vi "Main.vi"(11 "Module Admin":refnum<class "Delacor_lib_QMH_Module Admin.lvclass">) -> ()   [LabVIEW 2020, in "AO DC.lvlib"]
doc: "This template is based off of the Queued Message Handler design pattern and the Queued Message Handler project template that ships with LabVIEW.\n\nThe main difference is that the queue is private to this module and communication between modules is performed via Broadcast and Request events.\n\nRequest events are wrapped in public API methods and are handled in the Event Handling Loop (EHL) of this VI. Any module can register for Broadcast events sent by this module. The EHL generates messages based on user interface actions.\n\nThe Message Handling Loop (MHL) processes messages generated by the EHL, or by other messages. The messages are string values, so new messages can be added easily to the Message Cases case structure in the MHL. Each message cluster can also provide an optional value for Message Data, which is a variant that can be converted to whatever message-specific data is required.\n_____\nBased on DQMH Project Template 6.1.0.94."
uses:
  AO DC.lvlib
  <vilib>/Delacor/Delacor QMH/Libraries/Module Admin_class/Delacor_lib_QMH_Module Admin.lvclass
  Module Data--cluster.ctl
  <vilib>/Delacor/Delacor QMH/Libraries/Message Queue_class/Delacor_lib_QMH_Message Queue.lvclass/Delacor_lib_QMH_Message Queue.ctl
  Stop Argument--cluster.ctl
  <vilib>/Delacor/Delacor QMH/Libraries/Module Admin_class/Delacor_lib_QMH_Module Admin.lvclass/Delacor_lib_QMH_Module Admin.ctl
  AO DC Init Argument--cluster.ctl
  AO DC Start Argument--cluster.ctl
  <vilib>/Utility/miscctls.llb/LVPointTypeDef.ctl
  <vilib>/Delacor/Delacor QMH/Libraries/Message Queue_class/Delacor_lib_QMH_Enqueue Message (Single).vi
  <vilib>/Delacor/Delacor QMH/Libraries/Module Admin_class/Delacor_lib_QMH_Get External Launch.vi
  <vilib>/DAQmx/write.llb/DAQmx Write (Analog DBL 1Chan 1Samp).vi
  <vilib>/Utility/error.llb/Error Cluster From Error Code.vi
  <vilib>/DAQmx/miscellaneous.llb/DAQmx Fill In Error Info.vi
  <vilib>/ErrorRing/Error Ring.xnode
  <vilib>/Delacor/Delacor QMH/Libraries/Message Queue_class/Delacor_lib_QMH_Message Queue.lvclass
panel:
  out "error out":errorcluster
  out "Status":string
  in  "Simulate MHL Error":bool
  in  "Simulate EHL Error":bool
  # "Other QMH Modules communicate with this Module via its Public API (wrappers for its Request Events).\n\nThis Module communicates with other Modules via its Broadcast Events.\nAny module that wants to get these messages, just registers for this module's Broadcast events."
  # "This template is for the Delacor Modified Queued Message Handler design pattern.\n\nSee the block diagram for more information on how to use this template."
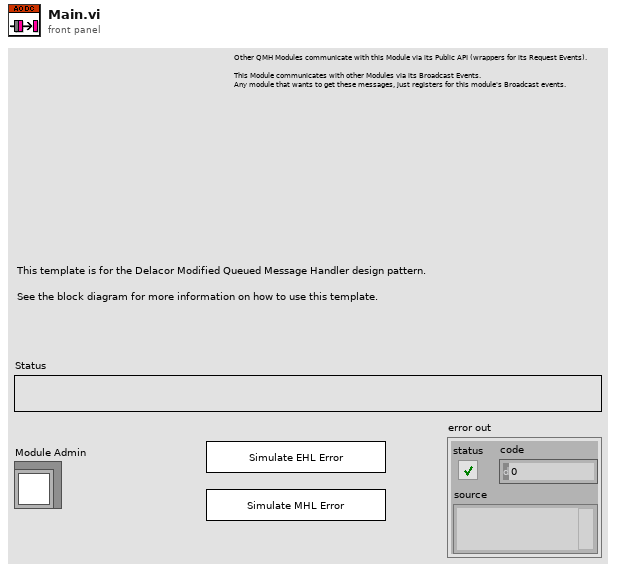
[diagram p1: front panel]
types:
  T1 = typedef "AO DC.lvlib/Request Events--cluster.ctl" = cluster{"Stop Module":refnum<user-event>, "Show Panel":refnum<user-event>, "Hide Panel":refnum<user-event>, "Get Module Execution Status":refnum<user-event>, "Show Diagram":refnum<user-event>, "AO DC Init":refnum<user-event>, "AO DC Start":refnum<user-event>}
  T2 = typedef "AO DC.lvlib/Module Data--cluster.ctl" = cluster{"Status":string, "AO DC Task":refnum<k21>, "User Value (Scaled)":dbl}
  T3 = enum32{"invalid lock state", "Not Locked", "Locked (No Password)", "Password-protected"}
  T4 = typedef "AO DC.lvlib/Stop Argument--cluster.ctl" = cluster{"Origin":string, "Exit via Stop Module Req?":bool, "Wait for Module to stop?":bool}
  T5 = typedef "AO DC.lvlib/AO DC Init Argument--cluster.ctl" = cluster{"AO DC Task":refnum<k21>, "User Value (Scaled)":dbl}
  T6 = typedef "AO DC.lvlib/AO DC Start Argument--cluster.ctl" = cluster{"Boolean":bool}
  T7 = typedef "LVPointTypeDef.ctl" = cluster{"Horizontal":i16, "Vertical":i16}
  T8 = enum32{"Invalid", "Standard", "Closed", "Hidden", "Minimized", "Maximized"}
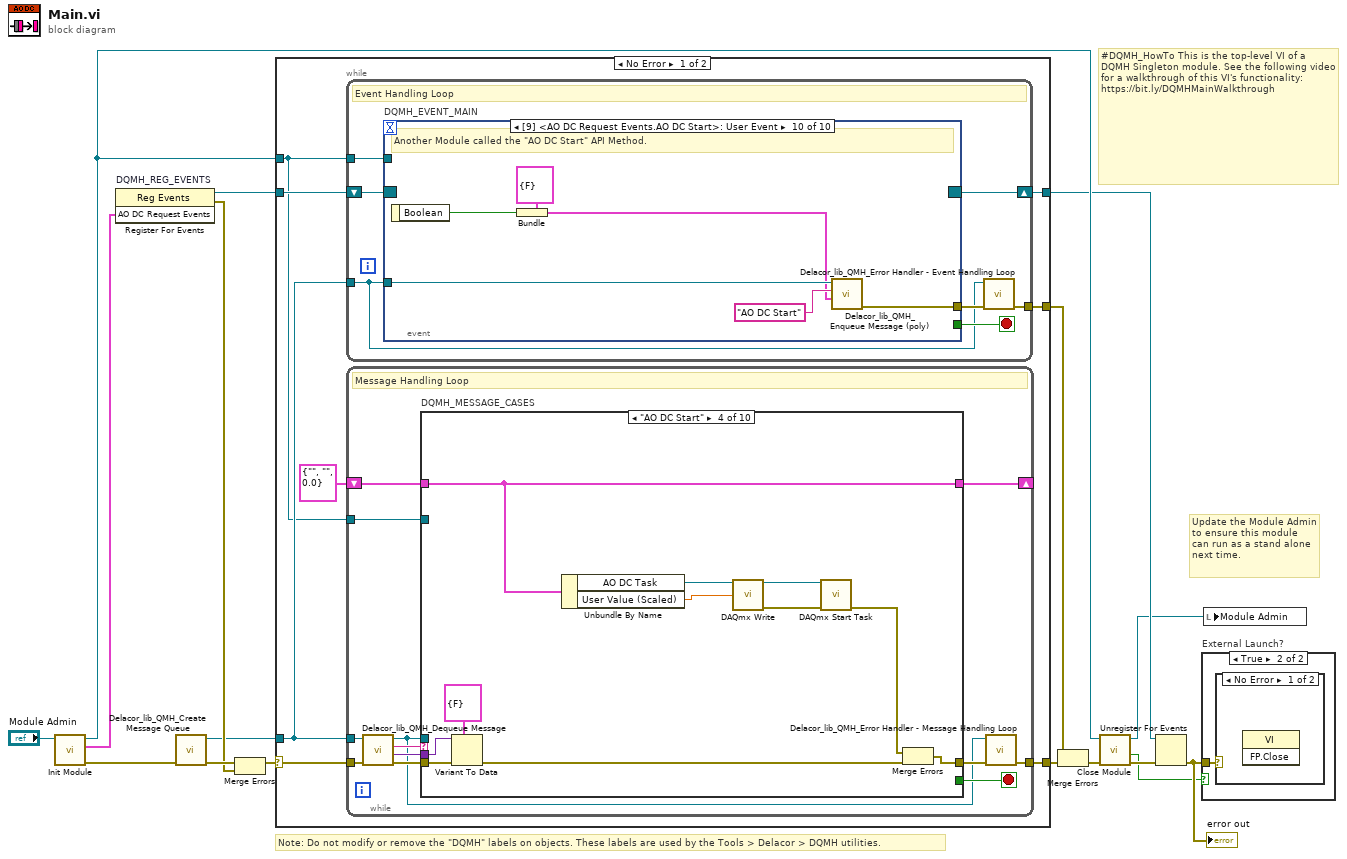
[diagram p0: block diagram]
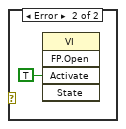
[diagram p3: hidden frame]
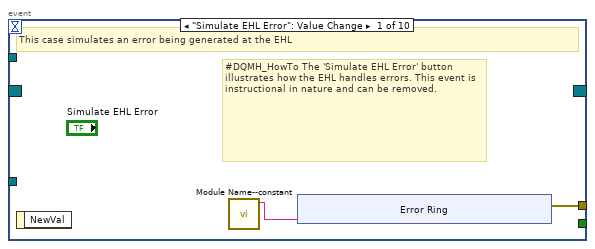
[diagram p4: hidden frame]
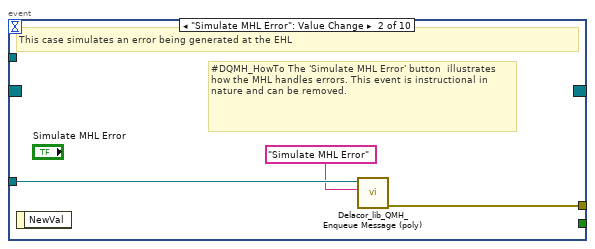
[diagram p5: hidden frame]
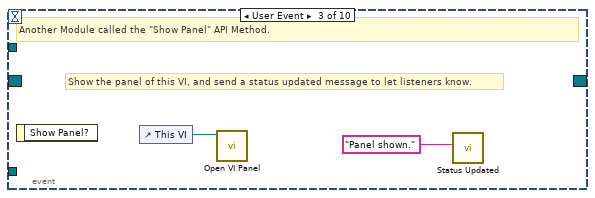
[diagram p6: hidden frame]
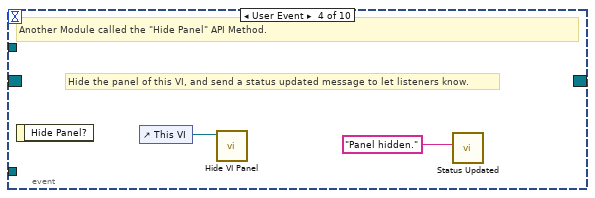
[diagram p7: hidden frame]
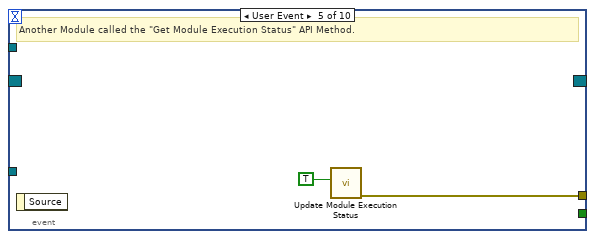
[diagram p8: hidden frame]
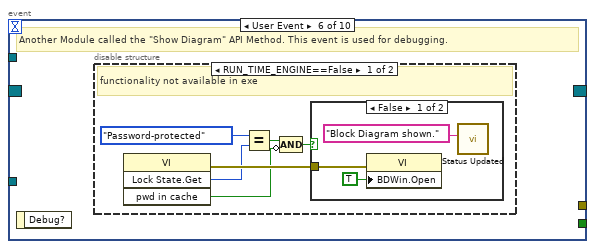
[diagram p9: hidden frame]
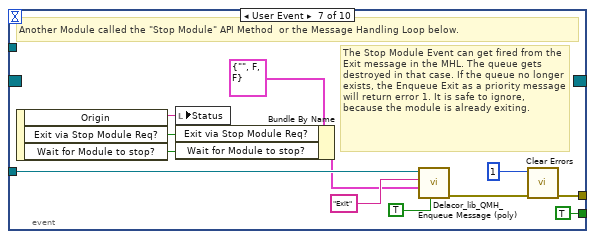
[diagram p12: hidden frame]
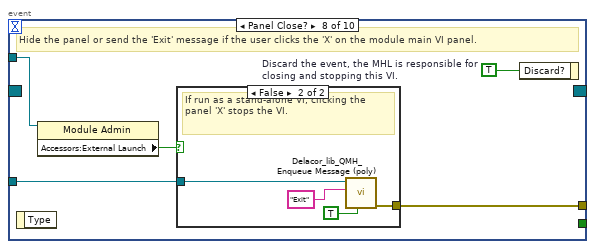
[diagram p13: hidden frame]
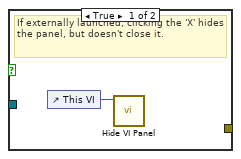
[diagram p14: hidden frame]
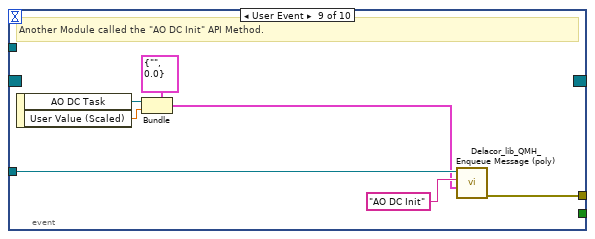
[diagram p15: hidden frame]
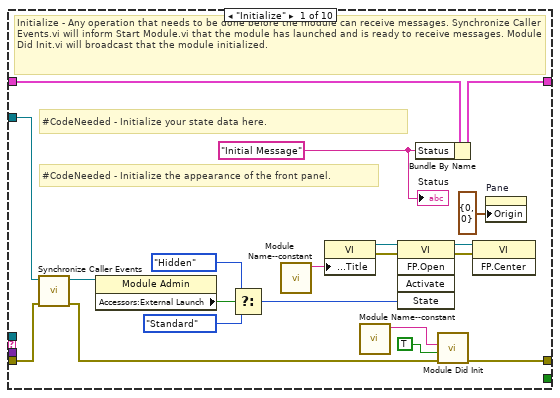
[diagram p16: hidden frame]
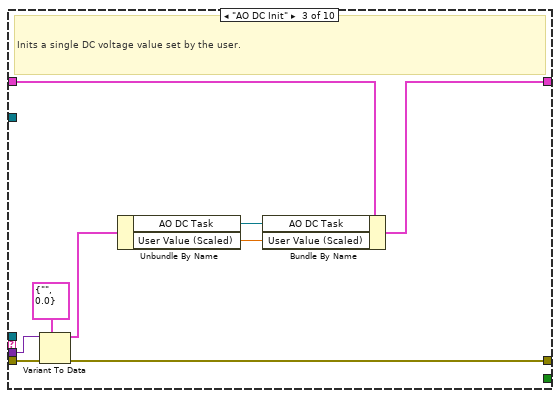
[diagram p18: hidden frame]
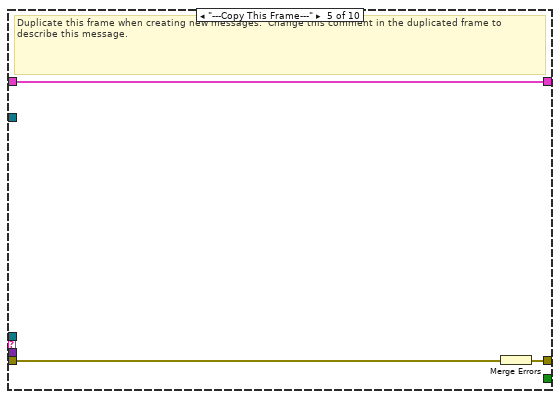
[diagram p19: hidden frame]
diagram:
  # "#DQMH_HowTo This is the top-level VI of a DQMH Singleton module. See the following video for a walkthrough of this VI's functionality: https://bit.ly/DQMHMainWalkthrough"
  # "Note: Do not modify or remove the \"DQMH\" labels on objects. These labels are used by the Tools > Delacor > DQMH utilities."
  # "Update the Module Admin to ensure this module can run as a stand alone next time."
  n1 = call "Init Module.vi"("Singleton Module Admin in"="Module Admin") -> ("error out"=w16:errorcluster, "AO DC Request Events"=w5:T1, "Singleton Module Admin out"=w8:refnum<class "Delacor_lib_QMH_Module Admin.lvclass">)  [unwired: 8 in]
  n2 = register-events "DQMH_REG_EVENTS"(w5) -> (reference out=w6:refnum<event-registration>, error out=w9:errorcluster)  [unwired: 2 in]
  n3 = call <vilib>:"Delacor_lib_QMH_Create Message Queue.vi"("error in"=w16) -> ("error out"=w11:errorcluster, "Message Queue"=w4:refnum<class "Delacor_lib_QMH_Message Queue.lvclass">)  [unwired: 9 in]
  n4 = Merge Errors(w11, w9) -> (w10:errorcluster)
  n5 = case shown="No Error" w10 {
    selector: w10 -> [w23 w213]
    tunnel: [w25 w212] -> w17
    tunnel: [w22 w218] -> w7
    tunnel: w6 -> [w20 w218]
    tunnel: w4 -> [w19 w211]
    tunnel: [w24 _] -> w14
    tunnel: w8 -> [w18 w214]
    frame No Error {
      n6 = while {
        tunnel: w19 -> [w26]
        shift-right: [w29] -> w22
        shift-left: w20 -> [w30]
        tunnel: [w31] -> w24
        tunnel: w18 -> [w27]
        stop <- w28 stop-if-true
        # "Event Handling Loop"
        n7 = event "DQMH_EVENT_MAIN" shown="[9] <AO DC Request Events.AO DC Start>: User Event" {
          selector: w30 -> [_ _ _ _ _ _ _ _ _ _]
          dyn-events: [_ _ _ _ _ _ _ _ _ _] -> w29
          timeout: _ -> [_ _ _ _ _ _ _ _ _ _]
          tunnel: [_ _ _ _ _ _ TRUE ("Discard?") _ _ _] -> w28
          tunnel: w26 -> [_ w43 _ _ _ _ w67 w74 w88 w94]
          tunnel: [w34 w44 _ _ w50 _ w70 w76 w82 w89] -> w32
          tunnel: w27 -> [_ _ _ _ _ _ _ w73 _ _]
          event "Simulate EHL Error": Value Change {
            # "#DQMH_HowTo The 'Simulate EHL Error' button  illustrates how the EHL handles errors. This event is instructional in nature and can be removed."
            # "This case simulates an error being generated at the EHL"
            n8 = event-data() -> ()  [unwired: 1 in, 1 out]
            n9 = call "Module Name--constant.vi"() -> ("Module Name"=w33:string)  [unwired: 11 in]
            n10 = xnode "Error Ring"("parameter 0"=w33) -> ("error out"=w34:errorcluster)
          }
          event "Simulate MHL Error": Value Change {
            # "#DQMH_HowTo The 'Simulate MHL Error' button  illustrates how the MHL handles errors. This event is instructional in nature and can be removed."
            # "This case simulates an error being generated at the EHL"
            n11 = event-data() -> ()  [unwired: 1 in, 1 out]
            n12 = call-poly <vilib>:"Delacor_lib_QMH_Enqueue Message (poly).vi"("Message"="Simulate MHL Error", "Message Queue in"=w43) -> ("error out"=w44:errorcluster)  [unwired: 8 in, 1 out]
          }
          event User Event {
            # "Show the panel of this VI, and send a status updated message to let listeners know."
            # "Another Module called the \"Show Panel\" API Method."
            n13 = event-data() -> ()  [unwired: 1 in, 1 out]
            n14 = control-ref of="This VI"() -> (w46:refnum<vi>)
            n15 = call "Open VI Panel.vi"("VI"=w46) -> ()  [unwired: 10 in, 1 out]
            n16 = call "Status Updated.vi"("Status"="Panel shown." ("format string")) -> ()  [unwired: 10 in, 1 out]
          }
          event User Event {
            # "Hide the panel of this VI, and send a status updated message to let listeners know."
            # "Another Module called the \"Hide Panel\" API Method."
            n17 = event-data() -> ()  [unwired: 1 in, 1 out]
            n18 = control-ref of="This VI"() -> (w48:refnum<vi>)
            n19 = call "Hide VI Panel.vi"("VI"=w48) -> ()  [unwired: 10 in, 1 out]
            n20 = call "Status Updated.vi"("Status"="Panel hidden." ("format string")) -> ()  [unwired: 10 in, 1 out]
          }
          event User Event {
            # "Another Module called the \"Get Module Execution Status\" API Method."
            n21 = event-data() -> ()  [unwired: 1 in, 1 out]
            n22 = call "Update Module Execution Status.vi"("Running?"=TRUE) -> ("error out"=w50:errorcluster)  [unwired: 10 in]
          }
          event User Event {
            # "Another Module called the \"Show Diagram\" API Method. This event is used for debugging."
            n23 = event-data() -> ()  [unwired: 1 in, 1 out]
            n24 = disable-structure shown="RUN_TIME_ENGINE==False" {
              frame condition #0 (active) {
                # "functionality not available in exe"
                n25 = invoke class="VI" method="Lock State.Get"() -> (error out=w56:errorcluster, "Get Lock State"=w55:T3, "pwd in cache"=w52:bool)  [unwired: 4 in, 1 out]
                n26 = Equal?(x=T3."Password-protected", y=w55) -> (x = y?=w53:bool)
                n27 = Compound Arithmetic op=AND(w53, invert w52) -> (w51:bool)
                n28 = case shown="False" w51 {
                  tunnel: w56 -> [w59 _]
                  frame False {
                    n29 = property class="VI"(error in=w59, "BDWin.Open"=TRUE ("Block Diagram Window:Open")) -> ()  [unwired: 1 in, 2 out]
                    n30 = call "Status Updated.vi"("Status"="Block Diagram shown." ("format string")) -> ()  [unwired: 10 in, 1 out]
                  }
                  frame True {
                    # "Password-protected VI, and the password is not in the cache. Do not show the diagram."
                  }
                }
              }
              frame condition #1 {
              }
            }
          }
          event User Event {
            # "The Stop Module Event can get fired from the Exit message in the MHL. The queue gets destroyed in that case. If the queue no longer exists, the Enqueue Exit as a priority message will return error 1. It is safe to ignore, because the module is already exiting."
            # "Another Module called the \"Stop Module\" API Method  or the Message Handling Loop below."
            n31 = event-data() -> ("Origin"=w66:string, "Exit via Stop Module Req?"=w62:bool, "Wait for Module to stop?"=w61:bool)  [unwired: 1 in]
            n32 = local write "Status"(w66) -> ()
            n33 = Bundle By Name(cluster=T4 {"Origin"="", "Exit via Stop Module Req?"=FALSE, "Wait for Module to stop?"=FALSE} ("Stop Argument"), "Exit via Stop Module Req?"=w62, "Wait for Module to stop?"=w61) -> (w60:T4)
            n34 = call-poly <vilib>:"Delacor_lib_QMH_Enqueue Message (poly).vi"("Priority Message? (F)"=TRUE, "Message Data"=w60, "Message"="Exit", "Message Queue in"=w67) -> ("error out"=w71:errorcluster)  [unwired: 6 in, 1 out]
            n35 = call <vilib>:"Clear Errors.vi"("error in (no error)"=w71, "specific error code to clear (0: all)"=1) -> ("error out"=w70:errorcluster)  [unwired: 4 in, 1 out]
          }
          event Panel Close? {
            w75 = TRUE  # Discard the event, the MHL is responsible for closing and stopping this VI.
            # "Hide the panel or send the 'Exit' message if the user clicks the 'X' on the module main VI panel."
            n36 = event-data() -> ()  [unwired: 1 in, 1 out]
            n37 = property class="Module Admin"(reference=w73) -> ("Accessors:External Launch"=w72:bool)  [unwired: 1 in, 2 out]
            n38 = case shown="False" w72 {
              tunnel: w74 -> [_ w80]
              tunnel: [_ w81] -> w76
              frame True {
                # "If externally launched, clicking the 'X' hides the panel, but doesn't close it."
                n39 = control-ref of="This VI"() -> (w77:refnum<vi>)
                n40 = call "Hide VI Panel.vi"("VI"=w77) -> ()  [unwired: 10 in, 1 out]
              }
              frame False {
                # "If run as a stand-alone VI, clicking the panel 'X' stops the VI."
                n41 = call-poly <vilib>:"Delacor_lib_QMH_Enqueue Message (poly).vi"("Priority Message? (F)"=TRUE, "Message"="Exit", "Message Queue in"=w80) -> ("error out"=w81:errorcluster)  [unwired: 7 in, 1 out]
              }
            }
            n42 = event-data("Discard?"=w75) -> ()  [unwired: 1 in, 1 out]
          }
          event User Event {
            # "Another Module called the \"AO DC Init\" API Method."
            n43 = event-data() -> ("AO DC Task"=w84:refnum<k21>, "User Value (Scaled)"=w83:dbl)  [unwired: 1 in]
            n44 = Bundle(cluster=T5 {"AO DC Task"="", "User Value (Scaled)"=0.0} ("AO DC Init Argument"), "AO DC Task"=w84, "User Value (Scaled)"=w83) -> (w85:T5)
            n45 = call-poly <vilib>:"Delacor_lib_QMH_Enqueue Message (poly).vi"("Message Data"=w85, "Message"="AO DC Init", "Message Queue in"=w88) -> ("error out"=w82:errorcluster)  [unwired: 7 in, 1 out]
          }
          event User Event {
            # "Another Module called the \"AO DC Start\" API Method."
            n46 = event-data() -> ("Boolean"=w90:bool)  [unwired: 1 in]
            n47 = Bundle(cluster=T6 {"Boolean"=FALSE} ("AO DC Start Argument"), "Boolean"=w90) -> (w91:T6)
            n48 = call-poly <vilib>:"Delacor_lib_QMH_Enqueue Message (poly).vi"("Message Data"=w91, "Message"="AO DC Start", "Message Queue in"=w94) -> ("error out"=w89:errorcluster)  [unwired: 7 in, 1 out]
          }
        }
        n49 = call-dynamic "Delacor_lib_QMH_Error Handler - Event Handling Loop.vi"("error in"=w32, "Message Queue in"=w26) -> ("dup error in"=w31:errorcluster)  [unwired: 8 in, 1 out]
      }
      n50 = while {
        tunnel: w19 -> [w97]
        shift-right: [w101] -> _
        shift-left: T2 {"Status"="", "AO DC Task"="", "User Value (Scaled)"=0.0} ("Data Cluster") -> [w102]
        tunnel: w23 -> [w105]
        tunnel: [w103] -> w25
        tunnel: w18 -> [w95]
        stop <- w100 stop-if-true
        # "Message Handling Loop"
        n51 = call-dynamic "Delacor_lib_QMH_Dequeue Message.vi"("error in"=w105, "Message Queue in"=w97) -> ("error out"=w104:errorcluster, "Message Data"=w98:variant, "Message"=w99:string, "Message Queue out"=w96:refnum<class "Delacor_lib_QMH_Message Queue.lvclass">)  [unwired: 6 in]
        n52 = case "DQMH_MESSAGE_CASES" shown="\"AO DC Start\"" w99 {
          selector: w99 -> [_ _ _ _ _ _ _ _ _ w198]
          tunnel: w96 -> [_ _ _ _ _ _ _ w168 w190 _]
          tunnel: w104 -> [w124 w128 w137 w148 w151 w153 w158 w175 w196 w200]
          tunnel: [w122 w128 w136 w140 w150 w153 w157 w171 w193 w201] -> w106
          tunnel: w102 -> [w113 w127 w132 w145 w149 w152 w155 w170 w189 w199]
          tunnel: [w112 w127 w130 w145 w149 w152 w155 w170 w189 w199] -> w101
          tunnel: [_ _ _ _ _ _ _ _ w188 _] -> w100
          tunnel: w98 -> [_ _ w135 w147 _ _ _ w169 w187 _]
          tunnel: w95 -> [w114 _ _ _ _ _ _ w167 w182 _]
          frame "Initialize" {
            w108 = "Initial Message" ("Initial Message")
            # "#CodeNeeded - Initialize the appearance of the front panel."
            # "#CodeNeeded - Initialize your state data here."
            # "Initialize - Any operation that needs to be done before the module can receive messages. Synchronize Caller Events.vi will inform Start Module.vi that the module has launched and is ready to receive messages. Module Did Init.vi will broadcast that the module initialized."
            n53 = call "Synchronize Caller Events.vi"("error in (no error)"=w124, "Singleton Module Admin in"=w114) -> ("error out"=w123:errorcluster, "Singleton Module Admin out"=w109:refnum<class "Delacor_lib_QMH_Module Admin.lvclass">)  [unwired: 8 in]
            n54 = property class="Module Admin"(reference=w109) -> ("Accessors:External Launch"=w118:bool)  [unwired: 1 in, 2 out]
            n55 = Select(t=T8."Hidden" ("State"), s=w118, f=T8."Standard" ("State")) -> (s? t:f=w115:T8)
            n56 = call "Module Name--constant.vi"() -> ("Module Name"=w121:string)  [unwired: 11 in]
            n57 = property class="VI"("Front Panel.Title"=w121) -> (reference out=w120:refnum<vi>, error out=w126:errorcluster)  [unwired: 2 in]
            n58 = call "Module Name--constant.vi"() -> ("Module Name"=w110:string)  [unwired: 11 in]
            n59 = invoke class="VI" method="FP.Open"(reference=w120, error in=w126, "State"=w115) -> (reference out=w119:refnum<vi>, error out=w125:errorcluster)  [unwired: 2 in, 3 out]
            n60 = Bundle By Name(cluster=w113, "Status"=w108) -> (w112:T2)
            n61 = call "Module Did Init.vi"("error in (no error)"=w123, "Initialized?"=TRUE, "Origin"=w110) -> ("error out"=w122:errorcluster)  [unwired: 8 in]
            n62 = invoke class="VI" method="FP.Center"(reference=w119, error in=w125) -> ()  [unwired: 1 in, 3 out]
            n63 = property on="Pane" class="Pane"("Origin"=T7 {"Horizontal"=0, "Vertical"=0}) -> ()  [unwired: 2 in, 2 out]
            "Status" <- w108
          }
          frame "---Module Specific---" {
            # "Separator -- The following cases handle messages specific to this Module."
          }
          frame "AO DC Init" {
            # "Inits a single DC voltage value set by the user."
            n64 = Variant To Data(error in=w137, type=T5 {"AO DC Task"="", "User Value (Scaled)"=0.0} ("AO DC Init Argument"), Variant=w135) -> (data=w133:T5, error out=w136:errorcluster)
            n65 = Unbundle By Name(w133) -> ("AO DC Task"=w131:refnum<k21>, "User Value (Scaled)"=w129:dbl)
            n66 = Bundle By Name(cluster=w132, "AO DC Task"=w131, "User Value (Scaled)"=w129) -> (w130:T2)
          }
          frame "AO DC Start" {
            n67 = Variant To Data(error in=w148, type=T6 {"Boolean"=FALSE} ("AO DC Start Argument"), Variant=w147) -> (error out=w139:errorcluster)  [unwired: 1 out]
            n68 = Unbundle By Name(w145) -> ("AO DC Task"=w144:refnum<k21>, "User Value (Scaled)"=w143:dbl)
            n69 = call-poly <vilib>:"DAQmx Write.vi"("task/channels in"=w144, "data"=w143) -> ("task out"=w142:refnum<k21>, "error out"=w141:errorcluster)  [unwired: 11 in, 1 out]
            n70 = call <vilib>:"DAQmx Start Task.vi"("task/channels in"=w142, "error in"=w141) -> ("error out"=w138:errorcluster)  [unwired: 12 in, 1 out]
            n71 = Merge Errors(w138, w139) -> (w140:errorcluster)
          }
          frame "---Copy This Frame---" {
            # "Duplicate this frame when creating new messages.  Change this comment in the duplicated frame to describe this message."
            n72 = Merge Errors(w151) -> (w150:errorcluster)
          }
          frame "---Exit and Error Handling---" {
            # "Separator - The following cases handle errors and exit messages."
          }
          frame "Simulate MHL Error" {
            # "#DQMH_HowTo The 'Simulate MHL Error' button  illustrates how the MHL handles errors. This event is instructional in nature and can be removed."
            # "Simulate an error occurring at the MHL"
            n73 = call "Module Name--constant.vi"() -> ("Module Name"=w154:string)  [unwired: 11 in]
            n74 = xnode "Error Ring"("parameter 0"=w154) -> ("error out"=w156:errorcluster)
            n75 = Merge Errors(w158, w156) -> (w157:errorcluster)
          }
          frame "Error" {
            # "#CodeRecommended - If you ever change the name of this \"Error\" message, you'll need to update the name in the Check Loop Error.vi as well."
            # "#CodeRecommended - If the module is running in standalone mode (External Launch = FALSE), this code will pop up an error dialog and call the 'Exit' message if an error occurs. Add more fine-grained error handling here."
            # "Error - Check the error message data and respond accordingly. This message is sent by the \"Error Handler\" VIs at the end of each loop in this application."
            n76 = property class="Module Admin"(reference=w167) -> ("Accessors:External Launch"=w166:bool)  [unwired: 1 in, 2 out]
            n77 = Variant To Data(error in=w175, type=errorcluster {"status"=FALSE, "code"=0, "source"=""} ("error constant"), Variant=w169) -> (data=w176:errorcluster, error out=w173:errorcluster)
            n78 = call "Error Reported.vi"("Error"=w176) -> ()  [unwired: 10 in, 1 out]
            n79 = case shown="False" w166 {
              tunnel: [w181 _] -> w172
              tunnel: w168 -> [w179 _]
              tunnel: w176 -> [w180 _]
              frame False {
                # "If the module is running standalone, then pop up an error dialog and call the \"Exit\" message."
                n80 = call <vilib>:"Simple Error Handler.vi"("error in (no error)"=w180) -> ()  [unwired: 4 in, 5 out]
                n81 = call-poly <vilib>:"Delacor_lib_QMH_Enqueue Message (poly).vi"("Priority Message? (F)"=TRUE, "Message"="Exit", "Message Queue in"=w179) -> ("error out"=w181:errorcluster)  [unwired: 7 in, 1 out]
              }
              frame True {
                # "If the module was launched externally, calling the Error Reported broadcast VI is the only action performed by the \"Error\" message. The module's caller can then process the error appropriately."
              }
            }
            n82 = Merge Errors(w173, w172) -> (w171:errorcluster)
            n83 = local write "error out"(w171) -> ()
          }
          frame "Exit" {
            w186 = 91  # 91: not all Exit messages will have an argument
            w188 = TRUE  # Stop the VI
            # "Release the message queue reference"
            # "#CodeNeeded - Add any required cleanup code here"
            # "Exit - Exit the application."
            n84 = Variant To Data(error in=w196, type=T4 {"Origin"="", "Exit via Stop Module Req?"=FALSE, "Wait for Module to stop?"=FALSE} ("Stop Argument"), Variant=w187) -> (data=w184:T4, error out=w192:errorcluster)
            n85 = call <vilib>:"Clear Errors.vi"("error in (no error)"=w192, "specific error code to clear (0: all)"=w186) -> ("error out"=w195:errorcluster)  [unwired: 4 in, 1 out]
            n86 = control-ref of="This VI"() -> (w183:refnum<vi>)
            n87 = call-dynamic "Delacor_lib_QMH_Release Message Queue.vi"("error in"=w195, "Message Queue"=w190) -> ("error out"=w194:errorcluster)  [unwired: 9 in]
            n88 = call "Handle Exit.vi"("Stop Argument"=w184, "Admin in"=w182, "VI reference"=w183) -> ("error out"=w191:errorcluster)  [unwired: 7 in, 1 out]
            n89 = Merge Errors(w194, w191) -> (w193:errorcluster)
          }
          frame Default {
            # "'Default' case only runs if there is a message that isn't defined in any of the other cases.  Output a programming error."
            n90 = call "Module Name--constant.vi"() -> ("Module Name"=w197:string)  [unwired: 11 in]
            n91 = xnode "Error Ring"("parameter 0"=w198, "parameter 1"=w197) -> ("error out"=w202:errorcluster)
            n92 = Merge Errors(w200, w202) -> (w201:errorcluster)
          }
        }
        n93 = call-dynamic "Delacor_lib_QMH_Error Handler - Message Handling Loop.vi"("error in"=w106, "Message Queue in"=w96) -> ("dup error in"=w103:errorcluster)  [unwired: 8 in, 1 out]
      }
    }
    frame Error {
      # "Synchronize Caller Events.vi will inform Start Module.vi that the module has launched and will let the code calling Start Module.vi register for broadcasts and would permit the caller receive the broadcast that an error occurred at launch time."
      n94 = call-dynamic "Delacor_lib_QMH_Release Message Queue.vi"("error in"=w213, "Message Queue"=w211) -> ("error out"=w212:errorcluster)  [unwired: 9 in]
      n95 = call "Synchronize Caller Events.vi"("Singleton Module Admin in"=w214) -> ("error out"=w219:errorcluster)  [unwired: 9 in, 1 out]
      n96 = call "Module Name--constant.vi"() -> ("Module Name"=w217:string)  [unwired: 11 in]
      n97 = Format Into String(format string="An error occurred during initialization. %s is no longer running.", w217) -> (resulting string=w215:string)  [unwired: 2 in, 1 out]
      n98 = Merge Errors(w212, w219) -> (w220:errorcluster)
      n99 = call "Error Reported.vi"("Additional Information"=w215, "Error"=w220) -> ()  [unwired: 9 in, 1 out]
    }
  }
  n100 = Merge Errors(w14, w17) -> (w13:errorcluster)
  n101 = call "Close Module.vi"("error in (no error)"=w13, "Module Admin in"=w8) -> ("error out"=w15:errorcluster, "External Launch"=w1:bool, "Module Admin out"=w2:refnum<class "Delacor_lib_QMH_Module Admin.lvclass">)  [unwired: 7 in]
  n102 = Unregister For Events(event registration refnum=w7, error in=w15) -> (error out=w12:errorcluster)
  "error out" <- w12
  n103 = case "External Launch?" shown="True" w1 {
    tunnel: w12 -> [_ w221]
    frame False {
    }
    frame True {
      n104 = case shown="No Error" w221 {
        frame No Error {
          n105 = invoke class="VI" method="FP.Close"() -> ()  [unwired: 3 in, 3 out]
        }
        frame Error {
          n106 = invoke class="VI" method="FP.Open"("Activate"=TRUE ("Activate?")) -> ()  [unwired: 4 in, 5 out]
        }
      }
    }
  }
  n107 = local write "Module Admin"(w2) -> ()
